vi "Pack for gRPC.vi"(8 "error in":errorcluster, 9 "configuration / results":enum16{"Configuration", "Results"}(ring), 10 "data value":variant, 11 "measurement plugin in":refnum<class "CAN-LIN Frame Generator.lvclass">) -> (0 "error out":errorcluster, 2 "any":T1, 3 "measurement plugin out":refnum<class "CAN-LIN Frame Generator.lvclass">)   [LabVIEW 2025, in "CAN-LIN Frame Generator.lvclass"]
uses:
  CAN-LIN Frame Generator.lvclass
  CAN-LIN Frame Generator.lvclass/CAN-LIN Frame Generator.ctl
  Measurement Configuration.ctl
  Measurement Results.ctl
  a6012965-5700-4384-8228-972e71b6560c.vi
  2eca732d-dbaa-43bf-a7dd-ede2da65bc1b.vi
  <vilib>/Plug-In SDKs/Measurements/Measurement Plugin Service/Measurement Plugin Service.lvclass
  CAN-LIN Frame Generator UI/Toggle.ctl
  CAN-LIN Frame Generator UI/XNET Frame Type CAN.ctl
  <vilib>/gRPC/LabVIEW gRPC Library/Shared/Any.ctl
  <vilib>/gRPC/LabVIEW gRPC Library/grpc-lvsupport-release.lvlib
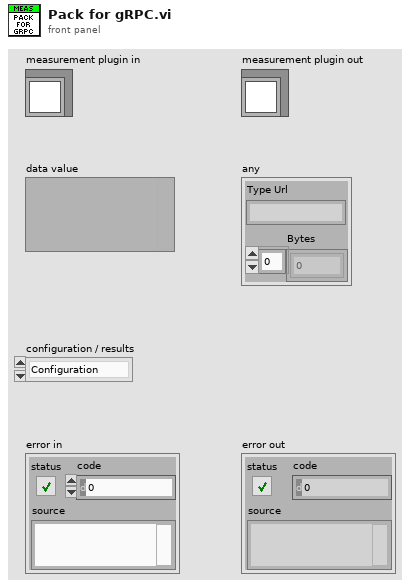
[diagram p1: front panel]
types:
  T1 = typedef "grpc-lvsupport-release.lvlib/Any.ctl" = cluster{"Type Url":string, "Bytes":u8[]}
  T2 = typedef "grpc-lvsupport-release.lvlib/grpcId.ctl" = u64
  T3 = typedef "CAN-LIN Frame Generator.lvclass/Measurement Configuration.ctl" = cluster{"INTERFACE NAME CAN":refnum<k21>, "IO Mode":enum32{"CAN", "CAN FD", "CAN FD + BRS"}, "FD ISO Mode":enum32{"ISO", "Legacy ISO", "Non-ISO"}, "Termination CAN":T4, "Baudrate":u32, "FD Baudrate":u32, "INTERFACE NAME LIN":refnum<k21>, "Termination LIN":T4, "CAN interface":string, "LIN interface":string, "IDENTIFIER":u32, "TYPE":T5, "DLC":u32, "SEND":bool, "PAYLOAD":u32[], "IDENTIFIER 2":u32, "DLC 2":u32, "SEND 2":bool, "PAYLOAD 2":u32[], "Tab No":string}
  T4 = typedef "Toggle.ctl" = bool
  T5 = typedef "XNET Frame Type CAN.ctl" = u32
  T6 = typedef "CAN-LIN Frame Generator.lvclass/Measurement Results.ctl" = cluster{"INTERFACE NAME CAN":refnum<k21>, "IO Mode":enum32{"CAN", "CAN FD", "CAN FD + BRS"}, "FD ISO Mode":enum32{"ISO", "Legacy ISO", "Non-ISO"}, "Baudrate":u32, "FD Baudrate":u32, "Termination CAN":T4, "INTERFACE NAME LIN":refnum<k21>, "Termination LIN":T4, "IDENTIFIER":u32, "TYPE":T5, "DLC":u32, "SEND":bool, "PAYLOAD":u32[], "IDENTIFIER 2":u32, "DLC 2":u32, "SEND 2":bool, "PAYLOAD 2":u32[]}
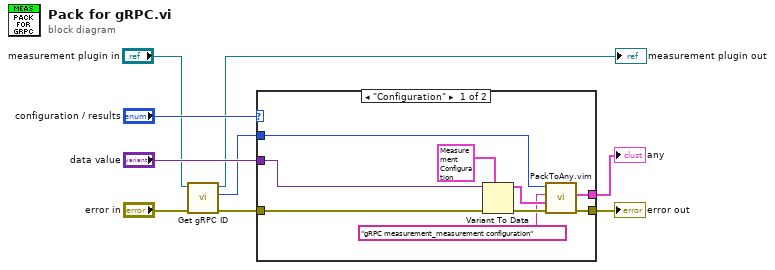
[diagram p0: block diagram]
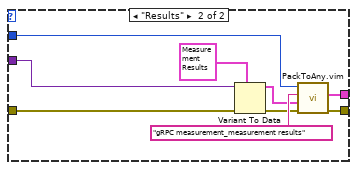
[diagram p2: hidden frame]
diagram:
  n1 = call <vilib>:"Get gRPC ID.vi"("error in"="error in", "measurement plugin service in"="measurement plugin in") -> ("error out"=w4:errorcluster, "gRPC ID"=w1:T2, "measurement plugin service out"=→"measurement plugin out":refnum<class "CAN-LIN Frame Generator.lvclass">)  [unwired: 7 in]
  n2 = case shown="\"Configuration\"" "configuration / results" {
    tunnel: w4 -> [w18 w27]
    tunnel: "data value" -> [w17 w26]
    tunnel: w1 -> [w14 w22]
    tunnel: [w16 w24] -> w8
    tunnel: [w15 w23] -> w7
    frame "Configuration" {
      n3 = Variant To Data(error in=w18, type=T3 {"INTERFACE NAME CAN"="Lorem ipsum dolor sit", "IO Mode"=enum."CAN FD", "FD ISO Mode"=enum."Non-ISO", "Termination CAN"=TRUE, "Baudrate"=64, "FD Baudrate"=64, "INTERFACE NAME LIN"="", "Termination LIN"=TRUE, "CAN interface"="", "LIN interface"="", "IDENTIFIER"=4294967264, "TYPE"=224, "DLC"=0, "SEND"=FALSE, "PAYLOAD"=[192, 191], "IDENTIFIER 2"=0, "DLC 2"=0, "SEND 2"=FALSE, "PAYLOAD 2"=[], "Tab No"=""} ("measurement configuration"), Variant=w17) -> (data=w13:T3, error out=w12:errorcluster)
      n4 = call "PackToAny.vim"("error in"=w12, "Data To Pack"=w13, "Message Type"="gRPC measurement_measurement configuration", "gRPCid in"=w14) -> ("error out"=w16:errorcluster, "Any"=w15:T1)  [unwired: 5 in, 1 out]
    }
    frame "Results" {
      n5 = Variant To Data(error in=w27, type=T6 {"INTERFACE NAME CAN"="Empty", "IO Mode"=enum."CAN", "FD ISO Mode"=enum."ISO", "Baudrate"=0, "FD Baudrate"=0, "Termination CAN"=FALSE, "INTERFACE NAME LIN"="", "Termination LIN"=FALSE, "IDENTIFIER"=0, "TYPE"=0, "DLC"=0, "SEND"=FALSE, "PAYLOAD"=[], "IDENTIFIER 2"=0, "DLC 2"=0, "SEND 2"=FALSE, "PAYLOAD 2"=[]} ("Measurement Results"), Variant=w26) -> (data=w20:T6, error out=w19:errorcluster)
      n6 = call "PackToAny.vim"("error in"=w19, "Data To Pack"=w20, "Message Type"="gRPC measurement_measurement results", "gRPCid in"=w22) -> ("error out"=w24:errorcluster, "Any"=w23:T1)  [unwired: 5 in, 1 out]
    }
  }
  "error out" <- w8
  "any" <- w7
